vi "End_Effector.vi"(2 "node":string, 5 "error in":errorcluster, 6 "Calibrate":bool caption="calibrate", 7 "Close":bool caption="Open", 8 "Side":T1) -> (0 "error out":errorcluster)   [LabVIEW 2013]
doc: "This will open or close the gripper to a specific position"
uses:
  ROS/Code/SubVIs/BaxterSide.ctl
  ROS/Code/_ROSDefinition.vi
  ROS/MessageBuilding/Primitives/subs/u32Scalar.vi
  ROS/MessageBuilding/Primitives/subs/stringScalar.vi
panel:
  out "msg out":string
  out "sequence":u32
  in  "No args":cluster{"args":string}
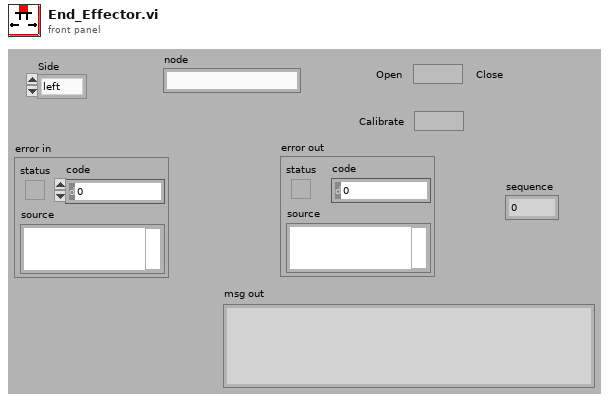
[diagram p1: front panel]
types:
  T1 = typedef "BaxterSide.ctl" = enum16{"left", "right"}
  T2 = cluster{"Seconds":u32, "NanoSec":u32, "ID":u32, "enabled":enum8{"FALSE", "TRUE", "UNKNOWN"}, "calibrated":enum8{"FALSE", "TRUE", "UNKNOWN"}, "ready":enum8{"FALSE", "TRUE", "UNKNOWN"}, "moving":enum8{"FALSE", "TRUE", "UNKNOWN"}, "gripping":enum8{"FALSE", "TRUE", "UNKNOWN"}, "missed":enum8{"FALSE", "TRUE", "UNKNOWN"}, "error":enum8{"FALSE", "TRUE", "UNKNOWN"}, "reverse":enum8{"FALSE", "TRUE", "UNKNOWN"}, "position":sgl, "force":sgl, "state":string, "command":string, "command sender":string, "command sequence":u32}
  T3 = typedef "_ROSControl.ctl" = cluster{"topic port":u16, "Node":string, "topic":string, "type":string, "node port":u32, "error ":errorcluster, "Direction":T4, "APIs":string[]}
  T4 = typedef "_ROSDirection.ctl" = enum16{"Node", "Publisher", "Subscriber", "Service Client"}
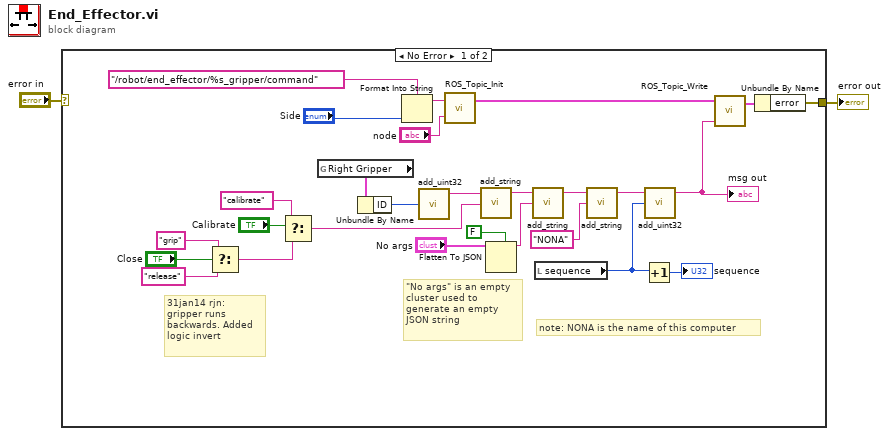
[diagram p0: block diagram]
diagram:
  n1 = case shown="No Error" "error in" {
    selector: "error in" -> [_ w30]
    tunnel: [w27 w30] -> w2
    frame No Error {
      # "31jan14 rjn:\ngripper runs \nbackwards. Added\nlogic invert"
      # "\"No args\" is an empty\ncluster used to \ngenerate an empty\nJSON string"
      # "note: NONA is the name of this computer"
      n2 = Select(t="grip", s="Close", f="release") -> (s? t:f=w5:string)
      n3 = Select(t="calibrate", s="Calibrate", f=w5) -> (s? t:f=w4:string)
      n4 = global read "_ROSDefinition.vi" "Right Gripper"() -> (w21:T2)
      n5 = Unbundle By Name(w21) -> ("ID"=w20:u32)
      n6 = Format Into String(format string="/robot/end_effector/%s_gripper/command" ("topic"), "Side") -> (resulting string=w25:string)  [unwired: 2 in, 1 out]
      n7 = call-poly "add_uint32.vi"("Numeric"=w20) -> ("msg out"=w23:string)  [unwired: 4 in]
      n8 = call "ROS_Topic_Init.vi"("node"="node", "topic"=w25) -> ("ROS out"=w29:T3)  [unwired: 1 in]
      n9 = call-poly "add_string.vi"("String"=w4, "msg in"=w23) -> ("msg out"=w19:string)  [unwired: 3 in]
      n10 = Flatten To JSON(enable LabVIEW extensions? (T)=FALSE, anything="No args") -> (JSON string=w16:string)  [unwired: 1 in, 1 out]
      n11 = call-poly "add_string.vi"("String"=w16, "msg in"=w19) -> ("msg out"=w15:string)  [unwired: 3 in]
      n12 = local read "sequence"() -> (w10:u32)
      n13 = call-poly "add_string.vi"("String"="NONA", "msg in"=w15) -> ("msg out"=w12:string)  [unwired: 3 in]
      n14 = Increment(x=w10) -> (x+1=→"sequence":u32)
      n15 = call-poly "add_uint32.vi"("Numeric"=w10, "msg in"=w12) -> ("msg out"=w11:string)  [unwired: 3 in]
      "msg out" <- w11
      n16 = call "ROS_Topic_Write.vi"("Msg in"=w11, "ROS in"=w29) -> ("ROS out"=w28:T3)  [unwired: 2 in]
      n17 = Unbundle By Name(w28) -> ("error"=w27:errorcluster)
    }
    frame Error {
    }
  }
  "error out" <- w2
